vi "GraphSetting Appearance (Wave).vi"(4 "FitControlToPane?":bool, 6 "コマンド":T1, 8 "error in (no error)":errorcluster caption="err(in)", 10 "外観(in)":T2, 11 "波形グラフref(in)":refnum<vi>) -> (0 "error out":errorcluster caption="err(out)", 2 "外観(out)":T2)   [LabVIEW 2016]
uses:
  TypeDef/GraphSetting Appearance.ctl
  TypeDef/GraphSetting Command.ctl
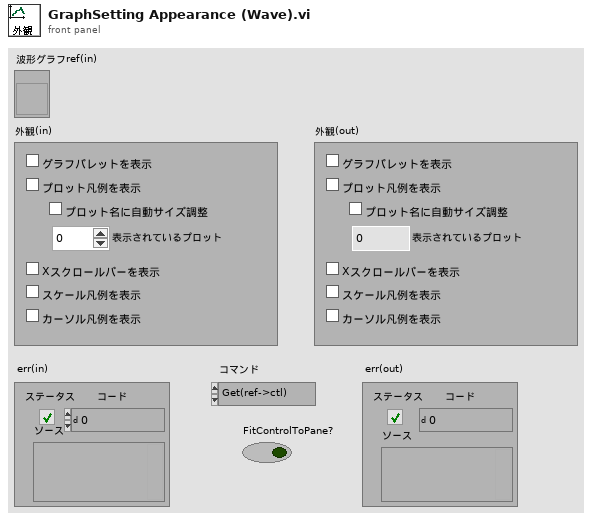
[diagram p1: front panel]
types:
  T1 = typedef "GraphSetting Command.ctl" = enum16{"Get(ref->ctl)", "Set(ctl->ref)"}
  T2 = typedef "GraphSetting Appearance.ctl" = cluster{"グラフパレットを表示":bool, "プロット凡例を表示":bool, "プロット名に自動サイズ調整":bool, "表示されているプロット":u32, "Xスクロールバーを表示":bool, "スケール凡例を表示":bool, "カーソル凡例を表示":bool}
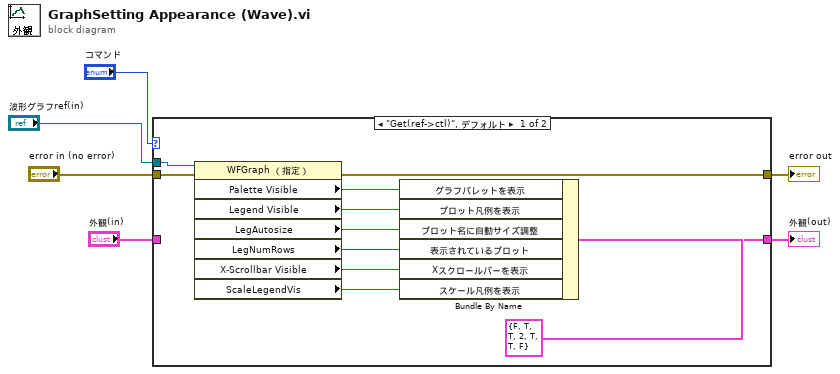
[diagram p0: block diagram]
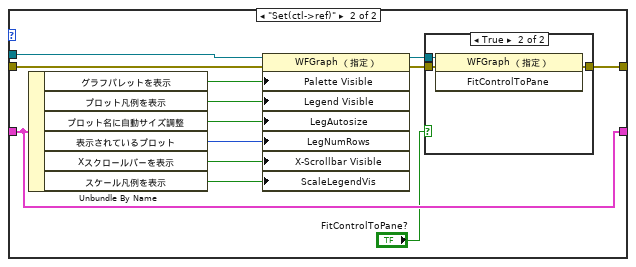
[diagram p2: hidden frame]
diagram:
  n1 = case shown="\"Get(ref->ctl)\", デフォルト" "コマンド" {
    tunnel: "波形グラフref(in)" -> [w10 w30]
    tunnel: [w9 w22] -> w6
    tunnel: "外観(in)" -> [_ w22]
    tunnel: "error in (no error)" -> [w8 w23]
    tunnel: [w7 w19] -> w2
    frame "Get(ref->ctl)", Default {
      n2 = property class="WFGraph （指定）"(reference=w10, error in=w8) -> (error out=w7:errorcluster, "Palette Visible"=w11:bool, "Legend Visible"=w12:bool, "LegAutosize"=w15:bool, "LegNumRows"=w16:u32, "X-Scrollbar Visible"=w13:bool, "ScaleLegendVis"=w14:bool)  [unwired: 1 out]
      n3 = Bundle By Name(cluster=T2 {"グラフパレットを表示"=FALSE, "プロット凡例を表示"=TRUE, "プロット名に自動サイズ調整"=TRUE, "表示されているプロット"=2, "Xスクロールバーを表示"=TRUE, "スケール凡例を表示"=TRUE, "カーソル凡例を表示"=FALSE} ("外観"), "グラフパレットを表示"=w11, "プロット凡例を表示"=w12, "プロット名に自動サイズ調整"=w15, "表示されているプロット"=w16, "Xスクロールバーを表示"=w13, "スケール凡例を表示"=w14) -> (w9:T2)
    }
    frame "Set(ctl->ref)" {
      n4 = Unbundle By Name(w22) -> ("グラフパレットを表示"=w24:bool, "プロット凡例を表示"=w25:bool, "プロット名に自動サイズ調整"=w26:bool, "表示されているプロット"=w27:u32, "Xスクロールバーを表示"=w28:bool, "スケール凡例を表示"=w29:bool)
      n5 = property class="WFGraph （指定）"(reference=w30, error in=w23, "Palette Visible"=w24, "Legend Visible"=w25, "LegAutosize"=w26, "LegNumRows"=w27, "X-Scrollbar Visible"=w28, "ScaleLegendVis"=w29) -> (reference out=w21:refnum<vi>, error out=w20:errorcluster)
      n6 = case shown="TRUE" "FitControlToPane?" {
        tunnel: w21 -> [_ w34]
        tunnel: w20 -> [w31 w33]
        tunnel: [w31 w32] -> w19
        frame False {
        }
        frame True {
          n7 = invoke class="WFGraph （指定）" method="FitControlToPane"(reference=w34, error in=w33) -> (error out=w32:errorcluster)  [unwired: 1 in, 2 out]
        }
      }
    }
  }
  "外観(out)" <- w6
  "error out" <- w2
